vi "Triggered Acquisition (Camera Link).vi"() -> ()   [LabVIEW 2023]
doc: "The Triggered Acquisition (Camera Link) example shows the basics of using a triggered acquisition by demonstrating how to configure the trigger settings."
uses:
  <vilib>/vision/driver/IMAQdx.llb/IMAQdx Buffer Number Mode.ctl
  <vilib>/vision/driver/IMAQdx.llb/IMAQdx Acquisition Mode.ctl
  <vilib>/vision/driver/NI_Vision_Acquisition_Software.lvlib
  <resource>/objmgr/imaqdx.rc
panel:
  in  "Trigger Parameters":T1={"Trigger Mode"=0, "Trigger Source"=65536, "Trigger Activation"=0, "Frame Timeout (ms)"=1000} {"Trigger Mode" items=["Off", "On"]; "Trigger Activation" items=["Rising Edge", "Falling Edge"]; "Trigger Source" items=["TTL 0"=65536, "TTL 1"=65537, "TTL 2"=65538, "TTL 3"=65539, "TTL 4"=65540, "TTL 5"=65541, "RTSI 0"=131072, "RTSI 1"=131073, "RTSI 2"=131074, "RTSI 3"=131075, "RTSI 4"=131076, "RTSI 5"=131077, "RTSI 6"=131078, "RTSI 7"=131079, "Iso In 0"=196608, "Iso In 1"=196609]}
  in  "Number of Images":i32=10
  in  "Camera Name":refnum<k21> caption="IMAQdx Session"
  out "Buffer Number":u32
  out "Image":T2(plugin-control)
  out "Frame Rate":dbl
  in  "Stop":bool
  # "Overview: Demonstrates how to dynamically enumerate the trigger sources and configure a triggered ring acquisition.\nRequirements: Vision Acquisition Software\nInstructions:\n1. Select the Camera Name and Number of Images. \n2. Run the VI\n3. Change the Trigger Parameters during run-time."
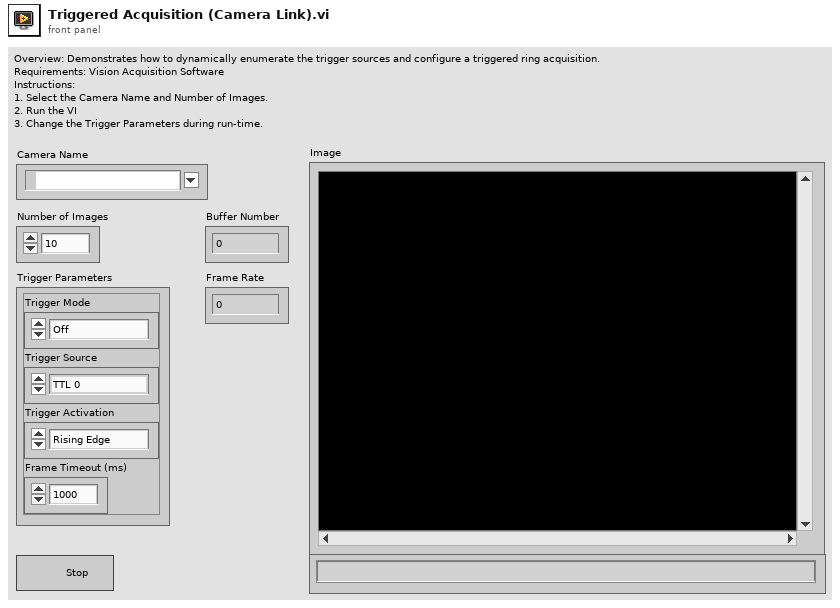
[diagram p1: front panel]
types:
  T1 = cluster{"Trigger Mode":u32, "Trigger Source":u32, "Trigger Activation":u32, "Frame Timeout (ms)":u32}
  T2 = typedef "IMAQ Image.ctl" = refnum<image>
  T3 = typedef "IMAQdx.ctl" = refnum<k21>
  T4 = typedef "NI_Vision_Acquisition_Software.lvlib/IMAQdx Buffer Number Mode.ctl" = enum32{"Next", "Last", "Buffer Number", "Every", "Last New"}
  T5 = typedef "NI_Vision_Acquisition_Software.lvlib/IMAQdx Acquisition Mode.ctl" = enum32{"One Shot", "Continuous"}
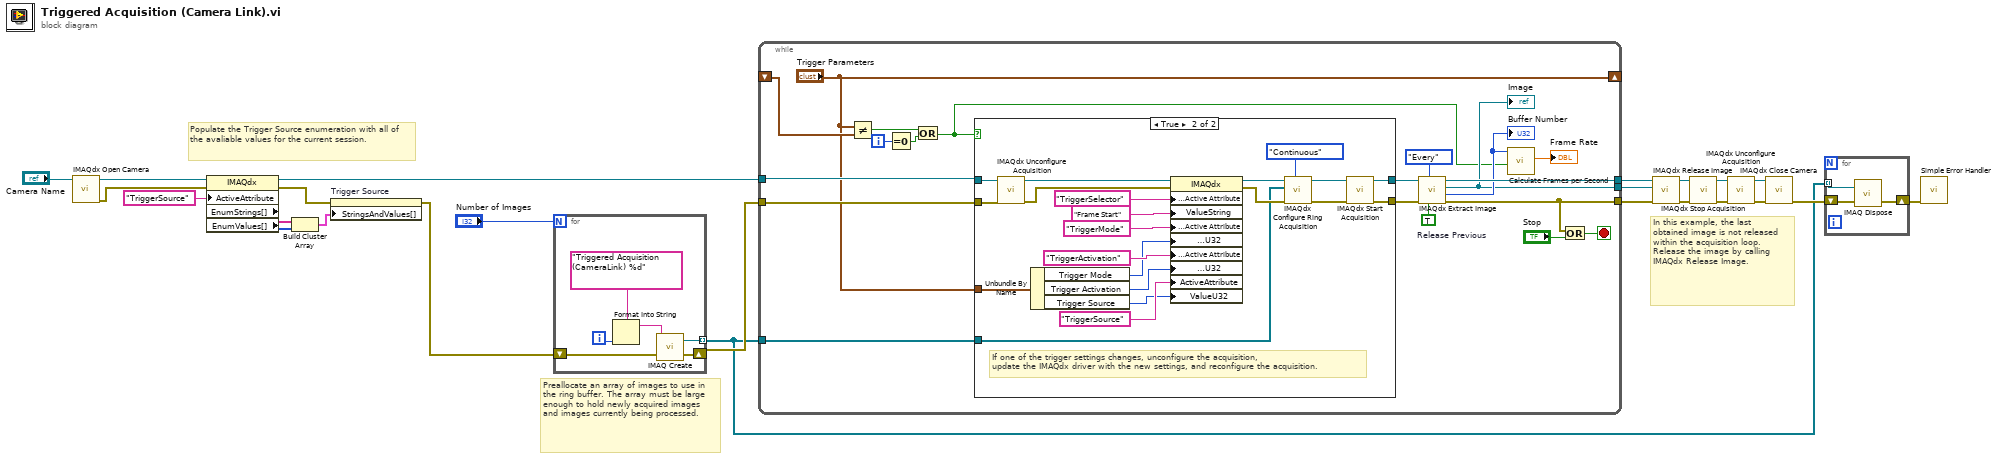
[diagram p0: block diagram]
diagram:
  # "Populate the Trigger Source enumeration with all of the avaliable values for the current session."
  # "Preallocate an array of images to use in the ring buffer. The array must be large enough to hold newly acquired images and images currently being processed."
  # "In this example, the last obtained image is not released within the acquisition loop. Release the image by calling IMAQdx Release Image."
  n1 = call <vilib>:"IMAQdx Open Camera.vi"("Session In"="Camera Name") -> ("error out"=w2:errorcluster, "Session Out"=w1:T3)  [unwired: 2 in, 7 out]
  n2 = property class="IMAQdx"(reference=w1, error in=w2, "ActiveAttribute"="TriggerSource") -> (reference out=w6:T3, error out=w8:errorcluster, "EnumStrings[]"=w11:string[], "EnumValues[]"=w10:u32[])
  n3 = Build Cluster Array(w11, w10) -> (w9:cluster{string, u32}[])
  n4 = property on="Trigger Source" class="Ring (strict)"(error in=w8, "StringsAndValues[]"=w9) -> (error out=w3:errorcluster)  [unwired: 1 in, 1 out]
  n5 = for {
    N: "Number of Images" -> [_]
    tunnel: [w29] -> w4 mode=indexing
    shift-right: [w28] -> w5
    shift-left: w3 -> [w30]
    i -> [w27]
    n6 = Format Into String(format string="Triggered Acquisition (CameraLink) %d" ("Image Name"), w27) -> (resulting string=w26:string)  [unwired: 2 in, 1 out]
    n7 = call "IMAQ Create"("Image Name"=w26, "error in (no error)"=w30) -> ("New Image"=w29:T2, "error out"=w28:errorcluster)  [unwired: 2 in, 1 out]
  }
  n8 = while {
    tunnel: [w49] -> w14
    tunnel: [w45] -> w16
    tunnel: [w42] -> w17
    shift-right: ["Trigger Parameters"] -> _
    shift-left: _ -> [w41]
    tunnel: w5 -> [w38]
    tunnel: w6 -> [w37]
    tunnel: w4 -> [w32]
    i -> [w31]
    stop <- w50 stop-if-true
    w43 = TRUE  # Release Previous
    n9 = Not Equal?(x="Trigger Parameters", y=w41) -> (x != y?=w39:bool)
    n10 = Equal To 0?(x=w31) -> (x = 0?=w40:bool)
    n11 = Or(x=w39, y=w40) -> (x .or. y?=w33:bool)
    n12 = case shown="True" w33 {
      tunnel: w38 -> [w51 w67]
      tunnel: w37 -> [w52 w66]
      tunnel: "Trigger Parameters" -> [_ w65]
      tunnel: [w52 w61] -> w35
      tunnel: [w51 w60] -> w34
      tunnel: w32 -> [_ w59]
      frame False {
      }
      frame True {
        # "If one of the trigger settings changes, unconfigure the acquisition, \nupdate the IMAQdx driver with the new settings, and reconfigure the acquisition."
        n13 = call <vilib>:"IMAQdx Unconfigure Acquisition.vi"("error in"=w67, "Session In"=w66) -> ("error out"=w72:errorcluster, "Session Out"=w73:T3)  [unwired: 8 out]
        n14 = Unbundle By Name(w65) -> ("Trigger Mode"=w55:u32, "Trigger Activation"=w54:u32, "Trigger Source"=w53:u32)
        n15 = property class="IMAQdx"(reference=w73, error in=w72, "Camera Attributes:Active Attribute"="TriggerSelector" ("ActiveAttribute"), "ValueString"="Frame Start", "Camera Attributes:Active Attribute"="TriggerMode" ("ActiveAttribute"), "Camera Attributes:Value:U32"=w55, "Camera Attributes:Active Attribute"="TriggerActivation" ("ActiveAttribute"), "Camera Attributes:Value:U32"=w54, "ActiveAttribute"="TriggerSource", "ValueU32"=w53) -> (reference out=w63:T3, error out=w62:errorcluster)
        n16 = call <vilib>:"IMAQdx Configure Ring Acquisition.vi"("Mode"=IMAQdx_Acquisition_Mode."Continuous" ("Continuous?"), "error in"=w62, "Images"=w59, "Session In"=w63) -> ("error out"=w70:errorcluster, "Session Out"=w69:T3)  [unwired: 5 in, 1 out]
        n17 = call <vilib>:"IMAQdx Start Acquisition.vi"("error in"=w70, "Session In"=w69) -> ("error out"=w60:errorcluster, "Session Out"=w61:T3)  [unwired: 8 out]
      }
    }
    n18 = call <vilib>:"IMAQdx Extract Image.vi"("Release Previous (true)"=w43, "Buffer Number Mode (Next)"=IMAQdx_Buffer_Number_Mode."Every" ("Buffer Number Mode"), "error in"=w34, "Session In"=w35) -> ("error out"=w45:errorcluster, "Buffer Number Out"=w46:u32, "Image Out"=w42:T2, "Session Out"=w49:T3)  [unwired: 4 in]
    "Image" <- w42
    "Buffer Number" <- w46
    n19 = call <vilib>:"Calculate Frames per Second.vi"("Reset"=w33, "Buffer Number"=w46) -> ("Processed Frames/s"=→"Frame Rate":dbl)  [unwired: 7 in, 2 out]
    n20 = Or(x=w45, y="Stop") -> (x .or. y?=w50:bool)
  }
  n21 = call <vilib>:"IMAQdx Release Image.vi"("error in"=w16, "Image"=w17, "Session In"=w14) -> ("error out"=w15:errorcluster, "Session Out"=w13:T3)  [unwired: 7 in]
  n22 = call <vilib>:"IMAQdx Stop Acquisition.vi"("error in"=w15, "Session In"=w13) -> ("error out"=w20:errorcluster, "Session Out"=w21:T3)  [unwired: 8 out]
  n23 = call <vilib>:"IMAQdx Unconfigure Acquisition.vi"("error in"=w20, "Session In"=w21) -> ("error out"=w23:errorcluster, "Session Out"=w22:T3)  [unwired: 8 out]
  n24 = call <vilib>:"IMAQdx Close Camera.vi"("error in"=w23, "Session In"=w22) -> ("error out"=w19:errorcluster)  [unwired: 9 out]
  n25 = for {
    shift-right: [w75] -> w18
    shift-left: w19 -> [w76]
    tunnel: w4 -> [w74] mode=indexing
    n26 = call "IMAQ Dispose"("Image"=w74, "error in (no error)"=w76) -> ("error out"=w75:errorcluster)  [unwired: 4 in]
  }
  n27 = call <vilib>:"Simple Error Handler.vi"("error in (no error)"=w18) -> ()  [unwired: 4 in, 5 out]
